vi "CThread Get Function Refnum By Name.vi"(0 "Name":string) -> (1 "Bounds":cluster{"Name":string, "Bounds":T1}[](array[cluster]), 2 "vi reference":refnum<vi>, 3 "Failed":bool)   [LabVIEW 2012, in "CThread.lvlib"]
uses:
  CThread.lvlib
  <vilib>/XNodeSupport/XNodeRect32.ctl
  <vilib>/XNodeSupport/XNodeInt.ctl
  Base/CThread Base - For Loop.vi
  Base/CThread Base - Get Execution State.vi
  Base/CThread Base - Do When Loop.vi
  Base/CThread Base - Get Iteration Index.vi
  Base/CThread Base - Set Conditional Terminal.vi
  Base/CThread Base - Set Selector Terminal.vi
  Base/CThread Base - Get Loop Count.vi
  <vilib>/XNodeSupport/NI_XNodeSupport.lvlib
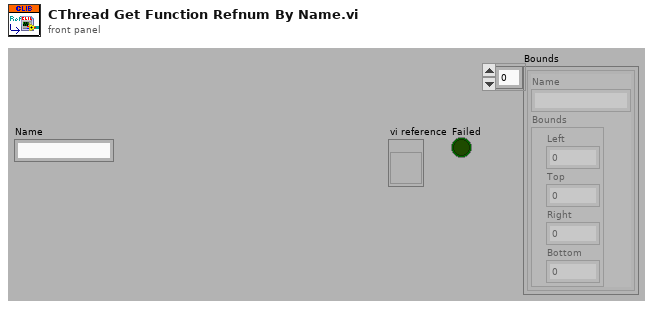
[diagram p1: front panel]
types:
  T1 = typedef "NI_XNodeSupport.lvlib/XNodeRect32.ctl" = cluster{"Left":T2, "Top":T2, "Right":T2, "Bottom":T2}
  T2 = typedef "NI_XNodeSupport.lvlib/XNodeInt.ctl" = i32
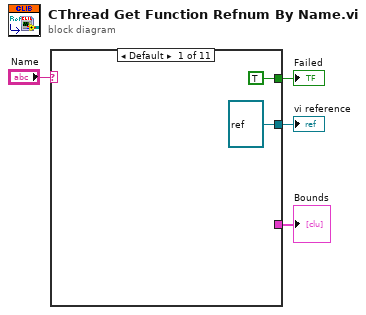
[diagram p0: block diagram]
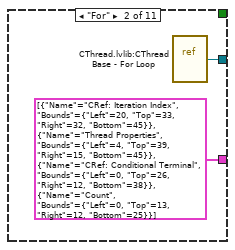
[diagram p2: hidden frame]
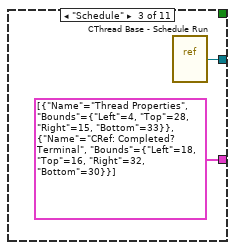
[diagram p3: hidden frame]
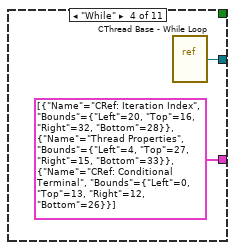
[diagram p4: hidden frame]
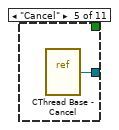
[diagram p5: hidden frame]
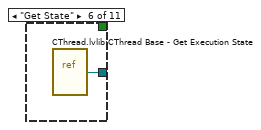
[diagram p6: hidden frame]
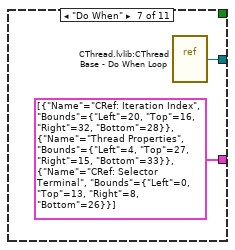
[diagram p7: hidden frame]
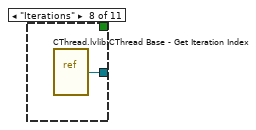
[diagram p8: hidden frame]
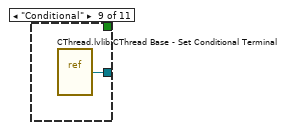
[diagram p9: hidden frame]
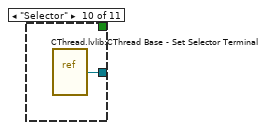
[diagram p10: hidden frame]
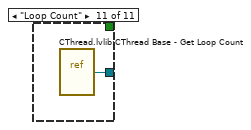
[diagram p11: hidden frame]
diagram:
  n1 = case shown="Default" "Name" {
    tunnel: [refnum<vi> refnum ("vi reference") w8 w10 w11 w13 w14 w15 w17 w18 w19 w20] -> w3
    tunnel: [TRUE _ _ _ _ _ _ _ _ _ _] -> w2
    tunnel: [_ cluster{"Name":string, "Bounds":T1}[] [{"Name"="CRef: Iteration Index", "Bounds"={"Left"=20, "Top"=33, "Right"=32, "Bottom"=45}}, {"Name"="Thread Properties", "Bounds"={"Left"=4, "Top"=39, "Right"=15, "Bottom"=45}}, {"Name"="CRef: Conditional Terminal", "Bounds"={"Left"=0, "Top"=26, "Right"=12, "Bottom"=38}}, {"Name"="Count", "Bounds"={"Left"=0, "Top"=13, "Right"=12, "Bottom"=25}}] ("Bounds") cluster{"Name":string, "Bounds":T1}[] [{"Name"="Thread Properties", "Bounds"={"Left"=4, "Top"=28, "Right"=15, "Bottom"=33}}, {"Name"="CRef: Completed? Terminal", "Bounds"={"Left"=18, "Top"=16, "Right"=32, "Bottom"=30}}] ("Bounds") cluster{"Name":string, "Bounds":T1}[] [{"Name"="CRef: Iteration Index", "Bounds"={"Left"=20, "Top"=16, "Right"=32, "Bottom"=28}}, {"Name"="Thread Properties", "Bounds"={"Left"=4, "Top"=27, "Right"=15, "Bottom"=33}}, {"Name"="CRef: Conditional Terminal", "Bounds"={"Left"=0, "Top"=13, "Right"=12, "Bottom"=26}}] ("Bounds") _ _ cluster{"Name":string, "Bounds":T1}[] [{"Name"="CRef: Iteration Index", "Bounds"={"Left"=20, "Top"=16, "Right"=32, "Bottom"=28}}, {"Name"="Thread Properties", "Bounds"={"Left"=4, "Top"=27, "Right"=15, "Bottom"=33}}, {"Name"="CRef: Selector Terminal", "Bounds"={"Left"=0, "Top"=13, "Right"=8, "Bottom"=26}}] ("Bounds") _ _ _ _] -> w1
    frame Default {
    }
    frame "For" {
      n2 = vi-ref "CThread.lvlib:CThread Base - For Loop.vi"() -> (w8:refnum<vi>)
    }
    frame "Schedule" {
      n3 = vi-ref "CThread Base - Schedule Run.vi"() -> (w10:refnum<vi>)
    }
    frame "While" {
      n4 = vi-ref "CThread Base - While Loop.vi"() -> (w11:refnum<vi>)
    }
    frame "Cancel" {
      n5 = vi-ref "CThread Base - Cancel.vi"() -> (w13:refnum<vi>)
    }
    frame "Get State" {
      n6 = vi-ref "CThread.lvlib:CThread Base - Get Execution State.vi"() -> (w14:refnum<vi>)
    }
    frame "Do When" {
      n7 = vi-ref "CThread.lvlib:CThread Base - Do When Loop.vi"() -> (w15:refnum<vi>)
    }
    frame "Iterations" {
      n8 = vi-ref "CThread.lvlib:CThread Base - Get Iteration Index.vi"() -> (w17:refnum<vi>)
    }
    frame "Conditional" {
      n9 = vi-ref "CThread.lvlib:CThread Base - Set Conditional Terminal.vi"() -> (w18:refnum<vi>)
    }
    frame "Selector" {
      n10 = vi-ref "CThread.lvlib:CThread Base - Set Selector Terminal.vi"() -> (w19:refnum<vi>)
    }
    frame "Loop Count" {
      n11 = vi-ref "CThread.lvlib:CThread Base - Get Loop Count.vi"() -> (w20:refnum<vi>)
    }
  }
  "vi reference" <- w3
  "Failed" <- w2
  "Bounds" <- w1
